vi "OffsetRect by V Array and Rect.vi"(8 "错误输入":errorcluster, 9 "V Array":i16[](array[numeric]), 11 "rect":T2 caption="矩形") -> (0 "错误输出":errorcluster, 3 "OffsetRect Array":T1(array[cluster]))   [LabVIEW 2012, in "Rect Tools.lvlib"]
uses:
  Rect Tools.lvlib
  OffsetRect by HV and Rect.vi
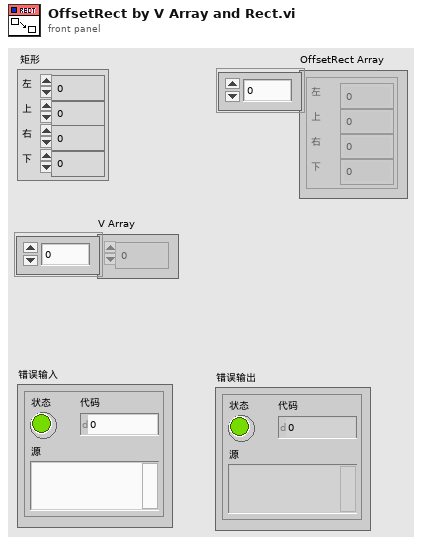
[diagram p1: front panel]
types:
  T1 = cluster{"left":i16, "top":i16, "right":i16, "bottom":i16}[]
  T2 = cluster{"left":i16, "top":i16, "right":i16, "bottom":i16}
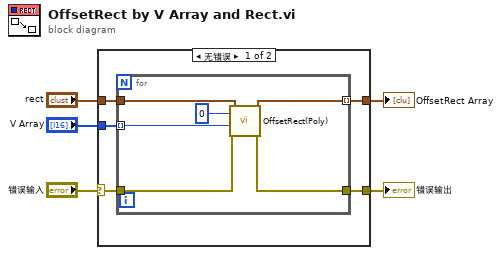
[diagram p0: block diagram]
diagram:
  n1 = case shown="无错误" "错误输入" {
    selector: "错误输入" -> [w7 w17]
    tunnel: [w6 w17] -> w4
    tunnel: "rect" -> [w10 _]
    tunnel: [w8 _] -> w1
    tunnel: "V Array" -> [w9 _]
    frame No Error {
      n2 = for {
        tunnel: w10 -> [w15]
        tunnel: w9 -> [w16] mode=indexing
        tunnel: [w14] -> w8 mode=indexing
        tunnel: w7 -> [w13]
        tunnel: [w12] -> w6
        n3 = call-poly "OffsetRect(Poly).vi"("错误输入"=w13, "v"=w16, "h"=i16 0, "rect"=w15) -> ("错误输出"=w12:errorcluster, "offset rect"=w14:T2)  [unwired: 6 in]
      }
    }
    frame Error {
    }
  }
  "错误输出" <- w4
  "OffsetRect Array" <- w1
